vi "ZScanRange.vi"(8 "error in (no error)":errorcluster, 11 "Z Scan Parameters":T1={"Z Range"=20.0, "Resolution"=1.0, "Initial Direction"=enum."Up", "Focus Threshold"=970.0, "Ascent Constant"=0.1} {"Focus Threshold" min=0.0 max=1000.0 step=1.0 format="%#_2f"; "Ascent Constant" min=0.0 max=1000.0 step=1.0 format="%#_2f"; "Resolution" min=0.0 max=1.0 step=0.01 format="%_2g"; "Z Range" format="%_3g"}) -> (0 "error out":errorcluster, 2 "Displacements":dbl[](array[numeric])=[0.0, 0.9523809523809524, 1.9047619047619049, 2.8571428571428568, 3.8095238095238098, 4.761904761904762, 5.7142857142857135, 6.666666666666667, 7.6190476190476195, 8.571428571428571, 9.523809523809524, 10.476190476190476, 11.428571428571427, 12.38095238095238, 13.333333333333334, 14.285714285714285, 15.238095238095239, 16.19047619047619, 17.142857142857142, 18.095238095238095, 19.047619047619047, 20.0, 19.047619047619047, 18.095238095238095, 17.142857142857146, 16.19047619047619, 15.238095238095239, 14.285714285714286, 13.333333333333332, 12.380952380952381, 11.42857142857143, 10.476190476190474, 9.523809523809524, 8.571428571428573, 7.619047619047622, 6.666666666666665, 5.714285714285714, 4.7619047619047645, 3.809523809523807, 2.8571428571428568, 1.904761904761906, 0.9523809523809554, -1.5265566588595902e-15, -0.9523809523809521, -1.9047619047619027, -2.857142857142853, -3.80952380952381, -4.761904761904761, -5.714285714285712, -6.666666666666669, -7.619047619047619, -8.57142857142857, -9.52380952380952, -10.476190476190478, -11.428571428571427, -12.380952380952378, -13.333333333333336, -14.285714285714286, -15.238095238095237, -16.190476190476186, -17.14285714285714, -18.095238095238088, -19.04761904761905, -19.999999999999996, -19.047619047619047, -18.095238095238095, -17.142857142857146, -16.190476190476197, -15.238095238095244, -14.285714285714281, -13.33333333333333, -12.38095238095238, -11.428571428571429, -10.47619047619048, -9.523809523809529, -8.571428571428578, -7.619047619047614, -6.666666666666664, -5.7142857142857135, -4.761904761904763, -3.809523809523812, -2.857142857142861, -1.9047619047619109, -0.9523809523809476, 0.0], 3 "Inspect?":bool[](array[boolean])=[TRUE, TRUE, TRUE, TRUE, TRUE, TRUE, TRUE, TRUE, TRUE, TRUE, TRUE, TRUE, TRUE, TRUE, TRUE, TRUE, TRUE, TRUE, TRUE, TRUE, TRUE, TRUE, TRUE, TRUE, TRUE, TRUE, TRUE, TRUE, TRUE, TRUE, TRUE, TRUE, TRUE, TRUE, TRUE, TRUE, TRUE, TRUE, TRUE, TRUE, TRUE, TRUE, TRUE, TRUE, TRUE, TRUE, TRUE, TRUE, TRUE, TRUE, TRUE, TRUE, TRUE, TRUE, TRUE, TRUE, TRUE, TRUE, TRUE, TRUE, TRUE, TRUE, TRUE, TRUE, TRUE, TRUE, TRUE, TRUE, TRUE, TRUE, TRUE, TRUE, TRUE, TRUE, TRUE, TRUE, TRUE, TRUE, TRUE, TRUE, TRUE, TRUE, TRUE, TRUE, TRUE])   [LabVIEW 2014]
uses:
  ZScan.ctl
  <vilib>/measure/NI_MABase.lvlib
panel:
  out "Displacements":waveform(dbl)(graph)={"t0"=timestamp(0 s since 1904-01-01), "dt"=0.011904761904761904, "Y"=[0.0, 0.9523809523809524, 1.9047619047619049, 2.8571428571428568, 3.8095238095238098, 4.761904761904762, 5.7142857142857135, 6.666666666666667, 7.6190476190476195, 8.571428571428571, 9.523809523809524, 10.476190476190476, 11.428571428571427, 12.38095238095238, 13.333333333333334, 14.285714285714285, 15.238095238095239, 16.19047619047619, 17.142857142857142, 18.095238095238095, 19.047619047619047, 20.0, 19.047619047619047, 18.095238095238095, 17.142857142857146, 16.19047619047619, 15.238095238095239, 14.285714285714286, 13.333333333333332, 12.380952380952381, 11.42857142857143, 10.476190476190474, 9.523809523809524, 8.571428571428573, 7.619047619047622, 6.666666666666665, 5.714285714285714, 4.7619047619047645, 3.809523809523807, 2.8571428571428568, 1.904761904761906, 0.9523809523809554, -1.5265566588595902e-15, -0.9523809523809521, -1.9047619047619027, -2.857142857142853, -3.80952380952381, -4.761904761904761, -5.714285714285712, -6.666666666666669, -7.619047619047619, -8.57142857142857, -9.52380952380952, -10.476190476190478, -11.428571428571427, -12.380952380952378, -13.333333333333336, -14.285714285714286, -15.238095238095237, -16.190476190476186, -17.14285714285714, -18.095238095238088, -19.04761904761905, -19.999999999999996, -19.047619047619047, -18.095238095238095, -17.142857142857146, -16.190476190476197, -15.238095238095244, -14.285714285714281, -13.33333333333333, -12.38095238095238, -11.428571428571429, -10.47619047619048, -9.523809523809529, -8.571428571428578, -7.619047619047614, -6.666666666666664, -5.7142857142857135, -4.761904761904763, -3.809523809523812, -2.857142857142861, -1.9047619047619109, -0.9523809523809476, 0.0]}
  # "LICENSED MATERIALS – PROPERTY OF IBM\nCopyright IBM Corp. 2016,\nALL RIGHTS RESERVED"
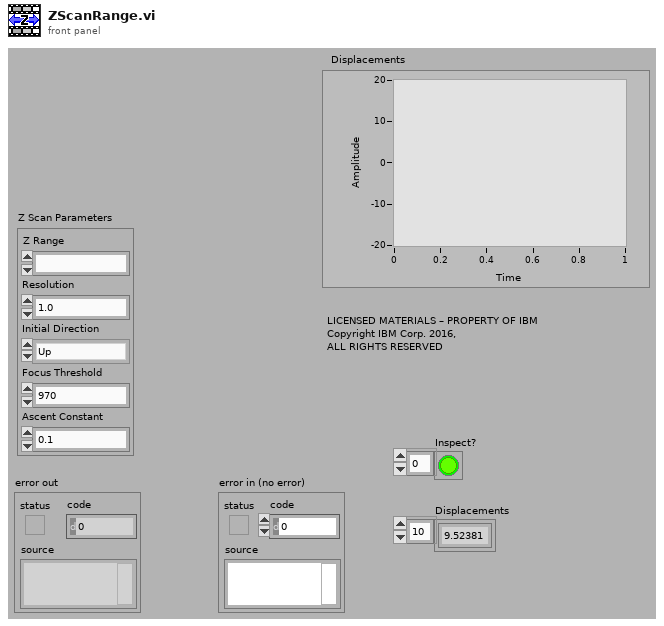
[diagram p1: front panel]
types:
  T1 = typedef "ZScan.ctl" = cluster{"Z Range":ext, "Resolution":dbl, "Initial Direction":enum16{"Up", "Down"}, "Focus Threshold":dbl, "Ascent Constant":dbl}
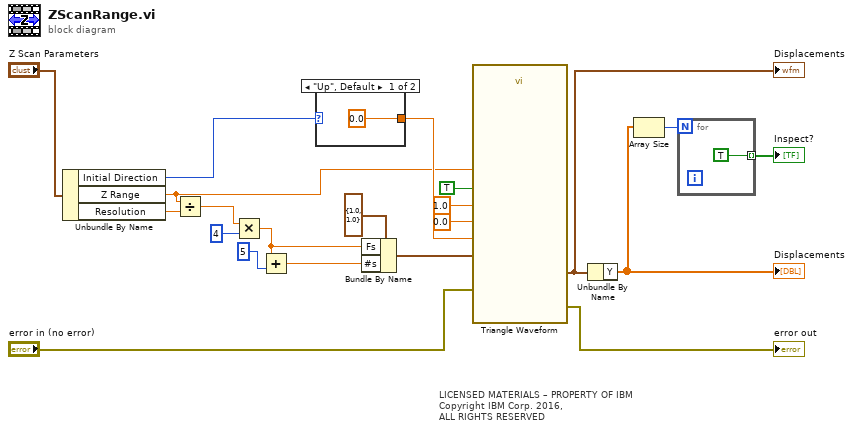
[diagram p0: block diagram]
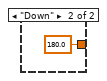
[diagram p2: hidden frame]
diagram:
  # "LICENSED MATERIALS – PROPERTY OF IBM\nCopyright IBM Corp. 2016,\nALL RIGHTS RESERVED"
  n1 = Unbundle By Name("Z Scan Parameters") -> ("Initial Direction"=w10:enum16{"Up", "Down"}, "Z Range"=w8:ext, "Resolution"=w7:dbl)
  n2 = Divide(x=w8, y=w7) -> (x/y=w6:ext)
  n3 = Multiply(x=w6, y=u32 4) -> (x*y=w2:ext)
  n4 = Add(x=w2, y=u32 5) -> (x+y=w12:ext)
  n5 = case shown="\"Up\", Default" w10 {
    tunnel: [0.0 ("offset") 180.0 ("offset")] -> w11
    frame "Up", Default {
    }
    frame "Down" {
    }
  }
  n6 = Bundle By Name(cluster=cluster{"Fs":dbl, "#s":dbl} {"Fs"=1.0, "#s"=1.0} ("sampling info 2"), "Fs"=w2, "#s"=w12) -> (w1:cluster{"Fs":dbl, "#s":dbl})
  n7 = call <vilib>:"Triangle Waveform.vi"("offset"=0.0, "sampling info"=w1, "reset signal"=TRUE, "error in (no error)"="error in (no error)", "phase"=w11, "amplitude"=w8, "frequency"=1.0 ("Fs")) -> ("error out"=→"error out":errorcluster, "signal out"=w9:waveform(dbl))  [unwired: 3 out]
  "Displacements" <- w9
  n8 = Unbundle By Name(w9) -> ("Y"=w5:dbl[])
  "Displacements" <- w5
  n9 = Array Size(array=w5) -> (size(s)=w4:i32)
  n10 = for {
    N: w4 -> [_]
    tunnel: [TRUE] -> w3 mode=indexing
  }
  "Inspect?" <- w3
